vi "MSEditor_Script_UpdateFunctionString.vi"(8 "error in (no error)":errorcluster, 10 "Func":string[](array[string]), 11 "Script of MS Process":refnum<vi>) -> (0 "error out":errorcluster)   [LabVIEW 2018]
uses:
  PublicSubVI/Class/DataXML/DataXML.lvclass
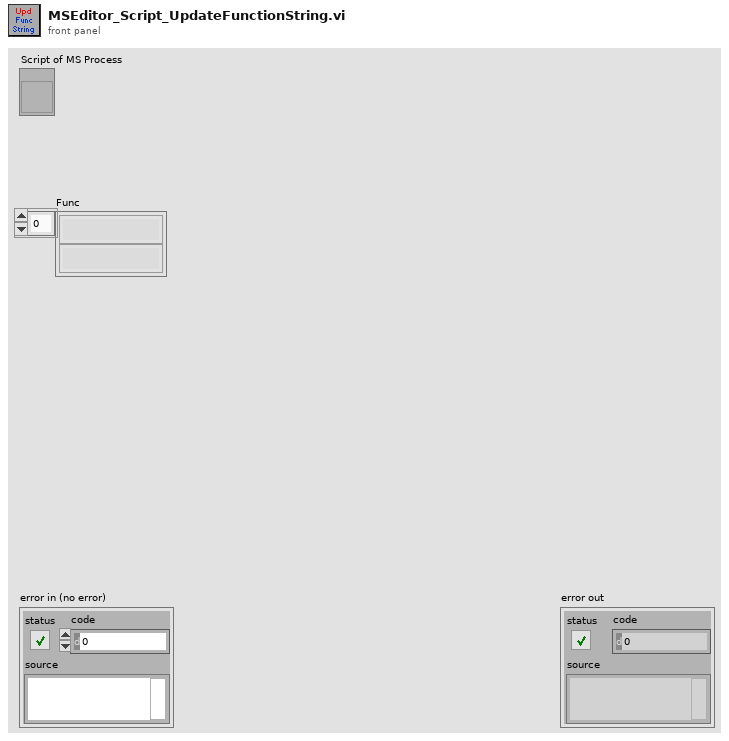
[diagram p1: front panel]
types:
  T1 = typedef "LVSelectionTypeDef.ctl" = cluster{"Selection Start":u32, "Selection End":u32}
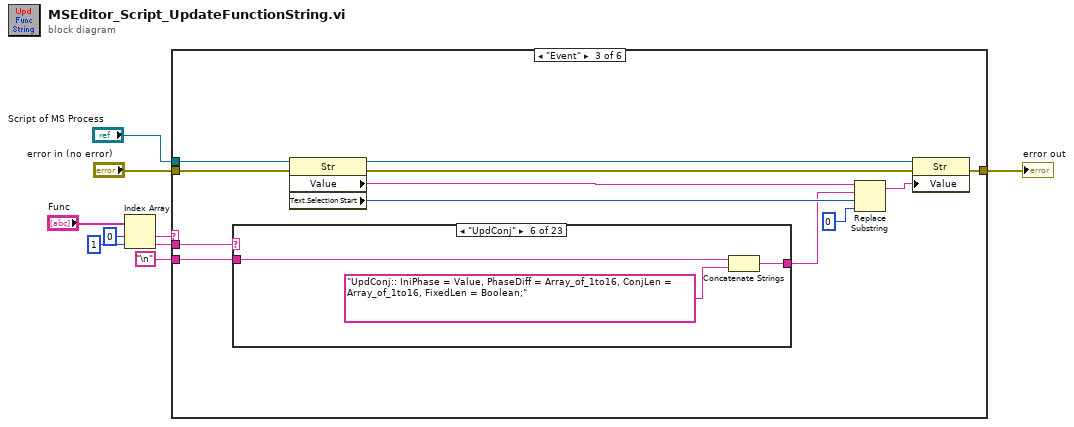
[diagram p0: block diagram]
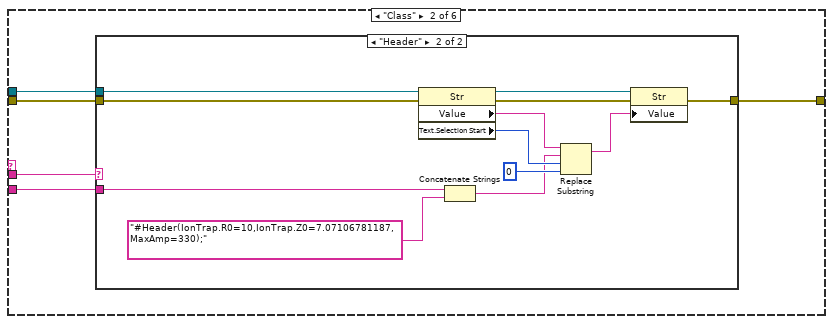
[diagram p3: hidden frame]
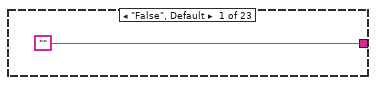
[diagram p5: hidden frame]
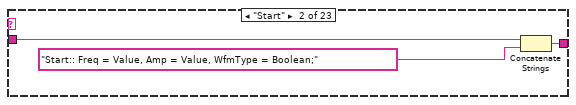
[diagram p6: hidden frame]
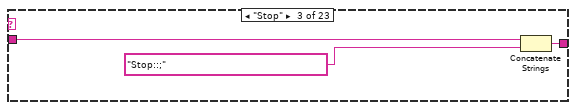
[diagram p7: hidden frame]
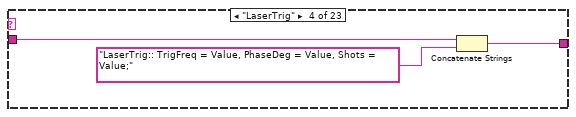
[diagram p8: hidden frame]
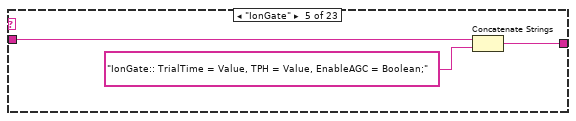
[diagram p9: hidden frame]
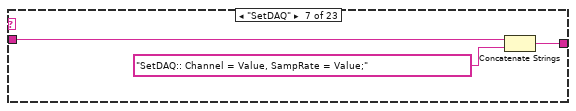
[diagram p10: hidden frame]
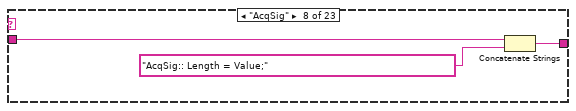
[diagram p11: hidden frame]
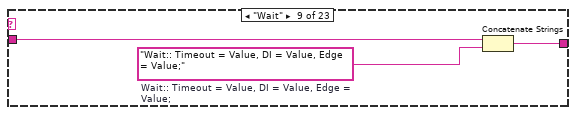
[diagram p12: hidden frame]
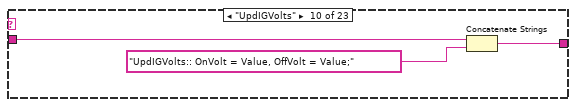
[diagram p13: hidden frame]
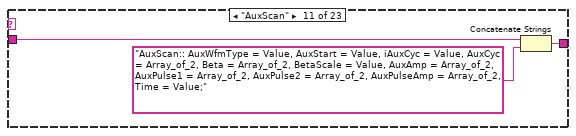
[diagram p14: hidden frame]
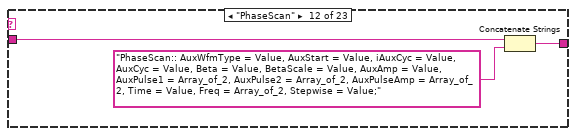
[diagram p15: hidden frame]
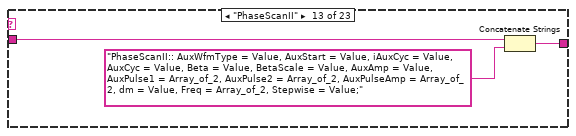
[diagram p16: hidden frame]
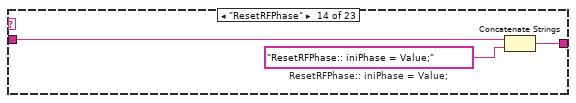
[diagram p17: hidden frame]
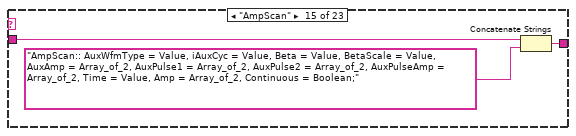
[diagram p18: hidden frame]
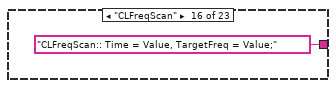
[diagram p19: hidden frame]
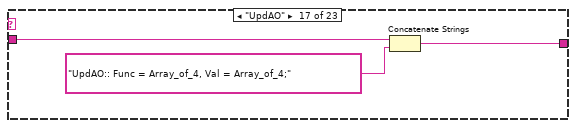
[diagram p20: hidden frame]
diagram:
  n1 = Index Array(array="Func", index #1=0 ("index"), index #2=1 ("index")) -> (element #1=w5:string, element #2=w4:string)
  n2 = case shown="\"Event\"" w5 {
    tunnel: "Script of MS Process" -> [_ w15 w40 w112 w170 w223]
    tunnel: "error in (no error)" -> [w10 w14 w39 w111 w169 w222]
    tunnel: w4 -> [_ w11 w30 w107 w167 w214]
    tunnel: "\n" -> [_ w13 w31 w110 w166 _]
    tunnel: [w10 w12 w29 w106 w168 w217] -> w1
    frame Default {
    }
    frame "Class" {
      n3 = case shown="\"Header\"" w11 {
        tunnel: w15 -> [_ w20]
        tunnel: w14 -> [w16 w19]
        tunnel: w13 -> [_ w18]
        tunnel: [w16 w17] -> w12
        frame Default {
        }
        frame "Header" {
          n4 = property class="Str"(reference=w20, error in=w19) -> (reference out=w28:refnum<vi>, error out=w27:errorcluster, "Value"=w24:string, "Text.Selection Start"=w25:u32)
          n5 = Concatenate Strings(w18, "#Header(IonTrap.R0=10,IonTrap.Z0=7.07106781187, MaxAmp=330);") -> (w23:string)
          n6 = Replace Substring(2:0 ("length (len. of substring)"), 3:w25, 4:w23, 5:w24) -> (1:w22:string)  [unwired: 1 out]
          n7 = property class="Str"(reference=w28, error in=w27, "Value"=w22) -> (error out=w17:errorcluster)  [unwired: 1 out]
        }
      }
    }
    frame "Event" {
      n8 = case shown="\"UpdConj\"" w30 {
        tunnel: w31 -> [_ w44 w47 w50 w53 w56 w59 w62 w64 w68 w71 w74 w77 w80 w83 _ w87 w90 w93 w95 w99 w102 w103]
        tunnel: ["" w43 w46 w49 w52 w54 w57 w60 w63 w67 w70 w73 w76 w79 w82 "CLFreqScan:: Time = Value, TargetFreq = Value;" w86 w89 w92 w94 w98 w101 w104] -> w33
        frame "False", Default {
        }
        frame "Start" {
          n9 = Concatenate Strings(w44, "Start:: Freq = Value, Amp = Value, WfmType = Boolean;") -> (w43:string)
        }
        frame "Stop" {
          n10 = Concatenate Strings(w47, "Stop::;") -> (w46:string)
        }
        frame "LaserTrig" {
          n11 = Concatenate Strings(w50, "LaserTrig:: TrigFreq = Value, PhaseDeg = Value, Shots = Value;") -> (w49:string)
        }
        frame "IonGate" {
          n12 = Concatenate Strings(w53, "IonGate:: TrialTime = Value, TPH = Value, EnableAGC = Boolean;") -> (w52:string)
        }
        frame "UpdConj" {
          n13 = Concatenate Strings(w56, "UpdConj:: IniPhase = Value, PhaseDiff = Array_of_1to16, ConjLen = Array_of_1to16, FixedLen = Boolean;") -> (w54:string)
        }
        frame "SetDAQ" {
          n14 = Concatenate Strings(w59, "SetDAQ:: Channel = Value, SampRate = Value;") -> (w57:string)
        }
        frame "AcqSig" {
          n15 = Concatenate Strings(w62, "AcqSig:: Length = Value;") -> (w60:string)
        }
        frame "Wait" {
          w65 = "Wait:: Timeout = Value, DI = Value, Edge = Value;"  # Wait:: Timeout = Value, DI = Value, Edge = Value;
          n16 = Concatenate Strings(w64, w65) -> (w63:string)
        }
        frame "UpdIGVolts" {
          n17 = Concatenate Strings(w68, "UpdIGVolts:: OnVolt = Value, OffVolt = Value;") -> (w67:string)
        }
        frame "AuxScan" {
          n18 = Concatenate Strings(w71, "AuxScan:: AuxWfmType = Value, AuxStart = Value, iAuxCyc = Value, AuxCyc = Array_of_2, Beta = Array_of_2, BetaScale = Value, AuxAmp = Array_of_2, AuxPulse1 = Array_of_2, AuxPulse2 = Array_of_2, AuxPulseAmp = Array_of_2, Time = Value;") -> (w70:string)
        }
        frame "PhaseScan" {
          n19 = Concatenate Strings(w74, "PhaseScan:: AuxWfmType = Value, AuxStart = Value, iAuxCyc = Value, AuxCyc = Value, Beta = Value, BetaScale = Value, AuxAmp = Value, AuxPulse1 = Array_of_2, AuxPulse2 = Array_of_2, AuxPulseAmp = Array_of_2, Time = Value, Freq = Array_of_2, Stepwise = Value;") -> (w73:string)
        }
        frame "PhaseScanII" {
          n20 = Concatenate Strings(w77, "PhaseScanII:: AuxWfmType = Value, AuxStart = Value, iAuxCyc = Value, AuxCyc = Value, Beta = Value, BetaScale = Value, AuxAmp = Value, AuxPulse1 = Array_of_2, AuxPulse2 = Array_of_2, AuxPulseAmp = Array_of_2, dm = Value, Freq = Array_of_2, Stepwise = Value;") -> (w76:string)
        }
        frame "ResetRFPhase" {
          w78 = "ResetRFPhase:: iniPhase = Value;"  # ResetRFPhase:: iniPhase = Value;
          n21 = Concatenate Strings(w80, w78) -> (w79:string)
        }
        frame "AmpScan" {
          n22 = Concatenate Strings(w83, "AmpScan:: AuxWfmType = Value, iAuxCyc = Value, Beta = Value, BetaScale = Value, AuxAmp = Array_of_2, AuxPulse1 = Array_of_2, AuxPulse2 = Array_of_2, AuxPulseAmp = Array_of_2, Time = Value, Amp = Array_of_2, Continuous = Boolean;") -> (w82:string)
        }
        frame "CLFreqScan" {
        }
        frame "UpdAO" {
          n23 = Concatenate Strings(w87, "UpdAO:: Func = Array_of_4, Val = Array_of_4;") -> (w86:string)
        }
        frame "UpdDO" {
          n24 = Concatenate Strings(w90, "UpdDO:: Func = Array_of_4, Val =  BooleanArray_of_4;") -> (w89:string)
        }
        frame "FGen" {
          n25 = Concatenate Strings(w93, "FGen:: Amp = Value, Freq = Value;") -> (w92:string)
        }
        frame "UpdRFChBias" {
          n26 = Concatenate Strings(w95, "UpdRFChBias:: ch1 = ext_value, ch2 = ext_value, ch3 = ext_value;") -> (w94:string)
        }
        frame "UpdRFChFunc" {
          n27 = Concatenate Strings(w99, "UpdRFChFunc:: ch1 = uint_value, ch2 = uint_value, ch3 = uint_value;\n%\n\nDefault. No output\n1. Pri\n2. OppPri\n3. Aux\n4. OppAux\n5. Pri+Aux\n6. Pri+OppAux\n7. OppPri+Aux\n8. OppPri+OppAux\n9. FGEN\n%") -> (w98:string)
        }
        frame "UpdRFChScale" {
          n28 = Concatenate Strings(w102, "UpdRFChScale:: ch1 = value, ch2 = value, ch3 = value;") -> (w101:string)
        }
        frame "UpdAuxArbPulses" {
          n29 = Concatenate Strings(w103, "UpdAuxArbPulses:: CycleIni = Array_of_1to255, CycleEnd = Array_of_1to255, PulseInt = Array_of_1to255;") -> (w104:string)
        }
      }
      n30 = property class="Str"(reference=w40, error in=w39) -> (reference out=w38:refnum<vi>, error out=w37:errorcluster, "Value"=w34:string, "Text.Selection Start"=w35:u32)
      n31 = Replace Substring(2:0 ("length (len. of substring)"), 3:w35, 4:w33, 5:w34) -> (1:w32:string)  [unwired: 1 out]
      n32 = property class="Str"(reference=w38, error in=w37, "Value"=w32) -> (error out=w29:errorcluster)  [unwired: 1 out]
    }
    frame "Calc" {
      n33 = case shown="\"Mathieu.mz\"" w107 {
        tunnel: w110 -> [_ w119 w122 w125 w128 w131 w134 w137 w140 w143 w146 w149 w152 w155 w158 w161 w164]
        tunnel: [_ w118 w121 w124 w127 w130 w133 w136 w139 w142 w145 w148 w151 w154 w157 w160 w163] -> w109
        frame Default {
        }
        frame "Add" {
          n34 = Concatenate Strings(w119, "#Calc(Add, r, a, b);\n% r = a + b %") -> (w118:string)
        }
        frame "Sub" {
          n35 = Concatenate Strings(w122, "#Calc(Sub, r, a, b);\n% r = a - b %") -> (w121:string)
        }
        frame "Times" {
          n36 = Concatenate Strings(w125, "#Calc(Times, r, a, b);\n%r = a * b %") -> (w124:string)
        }
        frame "Div" {
          n37 = Concatenate Strings(w128, "#Calc(Div, r, a, b);\n% r = a/b %") -> (w127:string)
        }
        frame "Pow" {
          n38 = Concatenate Strings(w131, "#Calc(Pow, r, a, b);\n% r = a^b %") -> (w130:string)
        }
        frame "Mod" {
          n39 = Concatenate Strings(w134, "#Calc(Mod, r, a, b);\n% r = a -floor(a/b)*b %") -> (w133:string)
        }
        frame "Floor" {
          n40 = Concatenate Strings(w137, "#Calc(Floor, r, a);\n% r = Floor(a) %") -> (w136:string)
        }
        frame "Ceil" {
          n41 = Concatenate Strings(w140, "#Calc(Ceil, r, a);\n% r = Ceil(a) %") -> (w139:string)
        }
        frame "Max" {
          n42 = Concatenate Strings(w143, "#Calc(Max, r, a, b);\n% r = Max(a, b) %") -> (w142:string)
        }
        frame "Min" {
          n43 = Concatenate Strings(w146, "#Calc(Min, r, a, b);\n% r = Min(a, b) %") -> (w145:string)
        }
        frame "Sign" {
          n44 = Concatenate Strings(w149, "#Calc(Sign, r, a);\n% r = Sign(a) %") -> (w148:string)
        }
        frame "Abs" {
          n45 = Concatenate Strings(w152, "#Calc(Abs, r, a);\n% r = Abs(a) %") -> (w151:string)
        }
        frame "Mathieu.mz" {
          n46 = Concatenate Strings(w155, "#Calc(Mathieu.mz, return, amp, freq, beta);\n%The function retruns a mz at condition parameters of amp, freq, and beta.   (a =0)%") -> (w154:string)
        }
        frame "Mathieu.beta" {
          n47 = Concatenate Strings(w158, "#Calc(Mathieu.beta, return, mz, amp, freq);") -> (w157:string)
        }
        frame "Mathieu.freq" {
          n48 = Concatenate Strings(w161, "#Calc(Mathieu.freq, return, mz, amp, beta);") -> (w160:string)
        }
        frame "Mathieu.amp" {
          n49 = Concatenate Strings(w164, "#Calc(Mathieu.amp, return, mz, freq, beta);") -> (w163:string)
        }
      }
      n50 = property class="Str"(reference=w112, error in=w111) -> (reference out=w117:refnum<vi>, error out=w116:errorcluster, "Value"=w114:string, "Text.Selection Start"=w115:u32)
      n51 = Replace Substring(2:0 ("length (len. of substring)"), 3:w115, 4:w109, 5:w114) -> (1:w108:string)  [unwired: 1 out]
      n52 = property class="Str"(reference=w117, error in=w116, "Value"=w108) -> (error out=w106:errorcluster)  [unwired: 1 out]
    }
    frame "Func" {
      n53 = case shown="\"IF\"" w167 {
        tunnel: w170 -> [_ w185 w190 w203]
        tunnel: w169 -> [w171 w184 w189 w202]
        tunnel: [w171 w172 w187 w200] -> w168
        tunnel: w166 -> [_ _ w188 w201]
        frame Default {
        }
        frame "Mark" {
          w173 = "%\n" ("substring (\"\")")
          w181 = 0 ("length (len. of substring)")
          n54 = property class="Str"(reference=w185, error in=w184) -> (reference out=w180:refnum<vi>, error out=w179:errorcluster, "Text.Selection"=w177:T1, "Value"=w183:string)
          n55 = Unbundle By Name(w177) -> ("Selection Start"=w186:u32, "Selection End"=w176:u32)
          n56 = Replace Substring(2:w181, 3:w176, 4:w173, 5:w183) -> (1:w182:string)  [unwired: 1 out]
          n57 = Increment(x=w176) -> (x+1=w175:u32)
          n58 = Replace Substring(2:w181, 3:w186, 4:w173, 5:w182) -> (1:w178:string)  [unwired: 1 out]
          n59 = Bundle By Name(cluster=w177, "Selection Start"=w175, "Selection End"=w175) -> (w174:T1)
          n60 = property class="Str"(reference=w180, error in=w179, "Text.Selection"=w174, "Value"=w178) -> (error out=w172:errorcluster)  [unwired: 1 out]
        }
        frame "Loop" {
          n61 = property class="Str"(reference=w190, error in=w189) -> (reference out=w199:refnum<vi>, error out=w198:errorcluster, "Value"=w196:string, "Text.Selection Start"=w197:u32)
          n62 = Concatenate Strings(w188, "#LoopStart(1);", w188, "#LoopEnd;") -> (w191:string)
          n63 = Replace Substring(2:0 ("length (len. of substring)"), 3:w197, 4:w191, 5:w196) -> (1:w195:string)  [unwired: 1 out]
          n64 = property class="Str"(reference=w199, error in=w198, "Value"=w195) -> (error out=w187:errorcluster)  [unwired: 1 out]
        }
        frame "IF" {
          n65 = property class="Str"(reference=w203, error in=w202) -> (reference out=w212:refnum<vi>, error out=w211:errorcluster, "Value"=w209:string, "Text.Selection Start"=w210:u32)
          n66 = Concatenate Strings(w201, "#If(value);", w201, "#IfEnd;") -> (w204:string)
          n67 = Replace Substring(2:0 ("length (len. of substring)"), 3:w210, 4:w204, 5:w209) -> (1:w208:string)  [unwired: 1 out]
          n68 = property class="Str"(reference=w212, error in=w211, "Value"=w208) -> (error out=w200:errorcluster)  [unwired: 1 out]
        }
      }
    }
    frame "User" {
      n69 = call <vilib>:"Application Directory.vi"() -> ("Application Directory"=w226:path)
      n70 = Build Path(base path=w226, name or relative path="instrument.ini") -> (appended path=w224:path)
      n71 = To Lower Case(string=w214) -> (all lower case string=w213:string)
      n72 = call "DataXML loadXmlProcess.vi"("xml_data_path"=w224) -> ("type"=w215:string[], "name"=w216:string[])  [unwired: 7 in, 2 out]
      n73 = To Lower Case(string=w216) -> (all lower case string=w221:string[])
      n74 = Equal?(x=w213, y=w221) -> (x = y?=w220:bool[])
      n75 = Search 1D Array(1D array=w220, element=TRUE) -> (index of element=w218:i32)  [unwired: 1 in]
      n76 = case shown="0, Default" w218 {
        selector: w218 -> [_ w236]
        tunnel: w223 -> [_ w244]
        tunnel: w222 -> [w227 w243]
        tunnel: [w227 w239] -> w217
        tunnel: w216 -> [_ w238]
        tunnel: w215 -> [_ w237]
        frame -1 {
        }
        frame 0, Default {
          n77 = Index Array(array=w238, index=w236) -> (element=w228:string)
          n78 = Index Array(array=w237, index=w236) -> (element=w235:string)
          n79 = Equal?(x=w235, y="array") -> (x = y?=w233:bool)
          n80 = Select(t="@" ("y"), s=w233, f="$" ("y")) -> (s? t:f=w229:string)
          n81 = property class="Str"(reference=w244, error in=w243) -> (reference out=w247:refnum<vi>, error out=w246:errorcluster, "Value"=w245:string, "Text.Selection Start"=w241:u32)
          n82 = Concatenate Strings(w229, w228) -> (w230:string)
          n83 = Replace Substring(2:0 ("length (len. of substring)"), 3:w241, 4:w230, 5:w245) -> (1:w242:string)  [unwired: 1 out]
          n84 = property class="Str"(reference=w247, error in=w246, "Value"=w242) -> (error out=w239:errorcluster)  [unwired: 1 out]
        }
      }
    }
  }
  "error out" <- w1
